vi "AO FGV.vi"(7 "Enum":enum16{"Read", "Write", "Start time", "init"}(ring), 9 "Start Time":timestamp, 10 "AO Channel Names":string[](array[string]), 11 "AO in":dbl[](array[numeric])) -> (1 "AO Waveform":waveform(dbl)[](array[waveform]), 3 "AO out":dbl[](array[numeric]))   [LabVIEW 2022 SP3]
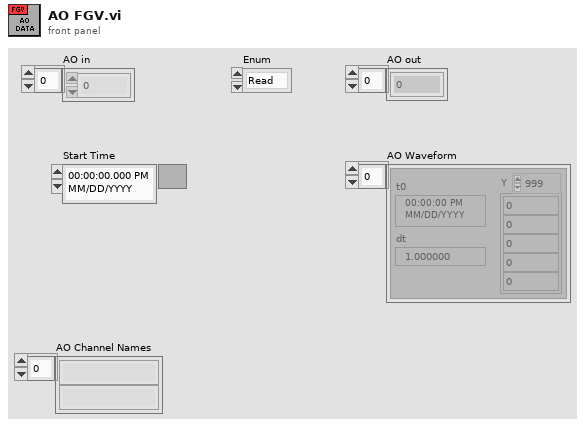
[diagram p1: front panel]
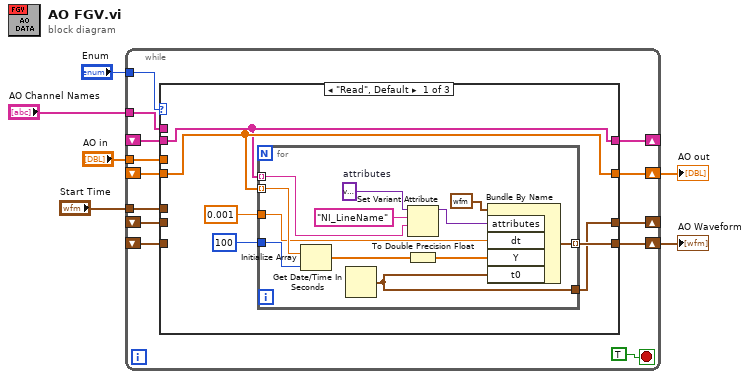
[diagram p0: block diagram]
diagram:
  n1 = while {
    tunnel: "Enum" -> [w18]
    tunnel: "AO in" -> [w17]
    shift-right: [w16] -> w3
    shift-left: _ -> [w15]
    tunnel: "Start Time" -> [w14]
    shift-right: [w13] -> _
    shift-left: _ -> [w12]
    shift-right: [w7] -> w4
    shift-left: _ -> [w11]
    shift-right: [w9] -> _
    shift-left: _ -> [w10]
    tunnel: "AO Channel Names" -> [w8]
    stop <- TRUE stop-if-true
    n2 = case shown="\"Read\", Default" w18 {
      tunnel: w17 -> [_ w41 _]
      tunnel: [w22 w41 w43] -> w16
      tunnel: w15 -> [w22 _ w43]
      tunnel: w14 -> [_ _ w45]
      tunnel: [w20 w40 w45] -> w13
      tunnel: w12 -> [_ w40 _]
      tunnel: [w23 w39 w44] -> w7
      tunnel: w11 -> [_ w39 w44]
      tunnel: w10 -> [w21 w38 _]
      tunnel: [w21 w38 w42] -> w9
      tunnel: w8 -> [_ _ w42]
      frame "Read", Default {
        n3 = for {
          tunnel: w22 -> [w36] mode=indexing
          tunnel: [w37] -> w23 mode=indexing
          tunnel: 100 ("Size") -> [w33]
          tunnel: w21 -> [w31] mode=indexing
          tunnel: 0.001 ("dt(sec)") -> [w28]
          tunnel: [w26] -> w20
          w32 = variant  # attributes
          n4 = Initialize Array(w36, w33) -> (w35:dbl[])
          n5 = Get Date/Time In Seconds() -> (seconds since 1Jan1904=w26:timestamp)
          n6 = Set Variant Attribute(Variant=w32, name="NI_LineName", value=w31) -> (Variant out=w27:variant)  [unwired: 1 in, 2 out]
          n7 = To Double Precision Float(number=w35) -> (double precision float=w34:dbl[])
          n8 = Bundle By Name(cluster=waveform(dbl) {"t0"=timestamp(0 s since 1904-01-01), "dt"=1.0, "Y"=[]} ("waveform"), "attributes"=w27, "dt"=w28, "Y"=w34, "t0"=w26) -> (w37:waveform(dbl))
        }
      }
      frame "Write" {
      }
      frame "Start time" {
      }
    }
  }
  "AO Waveform" <- w4
  "AO out" <- w3
